vi "FPGA.vi"() -> ()   [LabVIEW 2015]
doc: "This is the primary FPGA VI for the Build Your Own Embedded System project."
uses:
  Custom Controls/Battery State.ctl
  Custom Controls/Display State.ctl
  <vilib>/Platform/TimedLoop/XDataNode/timing_clust.ctl
  <vilib>/Platform/TimedLoop/XDataNode/nitl_modes.ctl
  <vilib>/Platform/TimedLoop/XDataNode/wakeup.ctl
  <vilib>/rvi/FXPMathLib/FxpDiv/subVIs/nifxpmath_Div_SimConfig.ctl
  <vilib>/rvi/Emulation/niFpgaGetClockAttributes.vi
  <vilib>/rvi/Emulation/niFpgaSctlEmulationGetInTimedLoop.vi
  <vilib>/rvi/Emulation/niFpgaEmulationReportErrorSimple.vi
  <vilib>/EmbeddedDisplay/Hitachi HD44780/FPGA/Internal/LCD Command.vi
  <vilib>/EmbeddedDisplay/Hitachi HD44780/FPGA/Public/Command Handler (8 Bits).vi
  <vilib>/rvi/Emulation/niFpgaProcessEmulError.vi
  <vilib>/rvi/Emulation/niFpgaCriticalErrorInLSC.vi
  <vilib>/rvi/eio/common/nirviEmuTemplateMethod_errors.vi
  <vilib>/rvi/Analysis/common/codeGenErrors/XNode/niFpgaXNodeCodeGenErrorHandle.vi
  <vilib>/rvi/Analysis/utilities/niFPGA Threshold Crossing Logic.vi
  <vilib>/rvi/FXPMathLib/FxpDiv/simVIs/DllFxpDivTemp_sub.vi
  <vilib>/eio/EIONode/EIONode.xnode
  <vilib>/rvi/Analysis/measure/period/templates/niFPGA Period Edge Direction.ctl
  <vilib>/rvi/Analysis/measure/period/XNode/niFpgaAnalogPeriod.xnode
  <vilib>/Platform/TimedLoop/XDataNode/XDataNode.xnode
  <vilib>/rvi/FXPMathLib/FxpDiv/XNode/nifxpmath_Div.xnode
  <vilib>/EmbeddedDisplay/Hitachi HD44780/FPGA/HD44780 FPGA.lvlib
  <vilib>/Platform/TimedLoop/XDataNode/XDNodeRunTimeDep.lvlib
panel:
  out "FPGA Display Command":T1=enum."RPM"
  out "Battery State":T2
  in  "Max Temp":fxp<+/-,32,13>
  out "Voltage":fxp<+/-,24,5>
  out "RPM":fxp<+,32,16>
  out "Temp":fxp<+/-,32,13>
  out "Temp Warning":bool
  in  "LCD Command":T3={"device index (-1)"=-1, "operation (0)"=0}
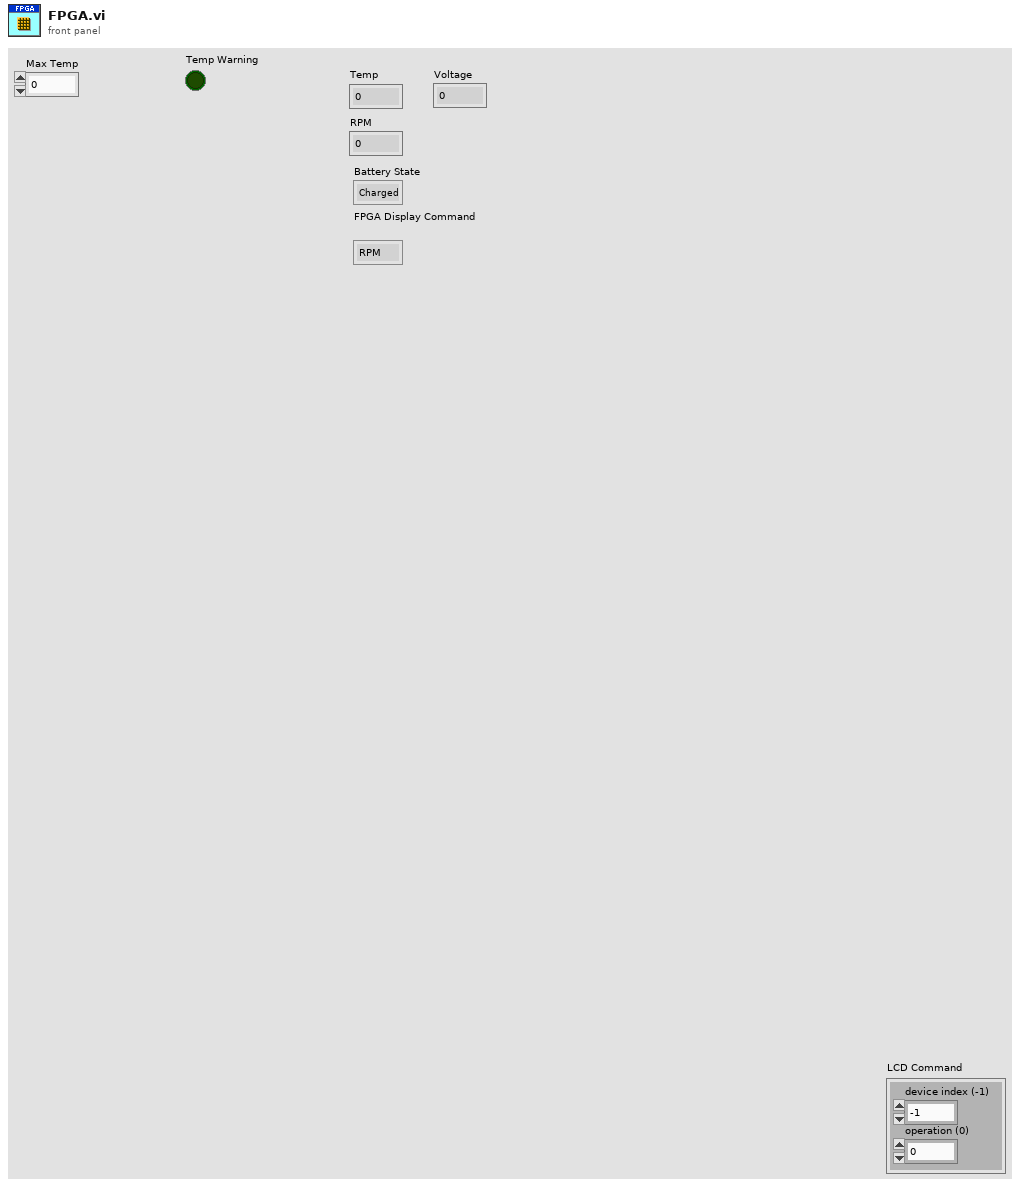
[diagram p1: front panel]
types:
  T1 = typedef "Display State.ctl" = enum16{"Battery State", "RPM", "Temp", "Voltage"}
  T2 = typedef "Battery State.ctl" = enum16{"Charged", "Running", "Low Batt"}
  T3 = cluster{"device index (-1)":i8, "operation (0)":u32}
  T4 = typedef "XDNodeRunTimeDep.lvlib/timing_clust.ctl" = cluster{"Expected End [f-1]":u64, "Actual End [f-1]":u64, "Finished Late? [f-1]":bool, "Expected End [i-1]":u64, "Actual End [i-1]":u64, "Finished Late? [i-1]":bool, "Expected Start [i]":u64, "Actual Start [i]":u64, "Expected Start [f]":u64, "Actual Start [f]":u64, "Source Name":string, "Structure Name":string, "Period":i64, "Deadline":i64, "Offset":i64, "Start":i64, "Priority":i32, "Timeout":i32, "Mode":T5, "Wakeup Reason":T6, "Error":errorcluster, "Source Type":string, "Secondary Source Type":string, "Global End Time":u64, "Global Start Time":u64, "Frame Duration":u64, "Iteration Duration":u64, "Assigned CPU":i32, "I/O Scan Engine Mode":u32}
  T5 = typedef "XDNodeRunTimeDep.lvlib/nitl_modes.ctl" = enum32{"No Change", "Process missed periods, maintain original phase", "Discard missed periods, maintain original phase", "Process missed periods, ignore original phase", "Discard missed periods, ignore original phase"}
  T6 = typedef "XDNodeRunTimeDep.lvlib/wakeup.ctl" = enum32{"Normal", "Aborted", "Asynchronous wakeup", "Timing source error", "Timed loop error", "Timeout"}
  T7 = cluster{"RS":refnum<k21>, "R/W":refnum<k21>, "E1":refnum<k21>, "E2":refnum<k21>, "DB0":refnum<k21>, "DB1":refnum<k21>, "DB2":refnum<k21>, "DB3":refnum<k21>, "DB4":refnum<k21>, "DB5":refnum<k21>, "DB6":refnum<k21>, "DB7":refnum<k21>}
  T8 = typedef "HD44780 Common.lvlib/lcd command cluster.ctl" = cluster{"device index (-1)":i8, "operation (0)":u32}
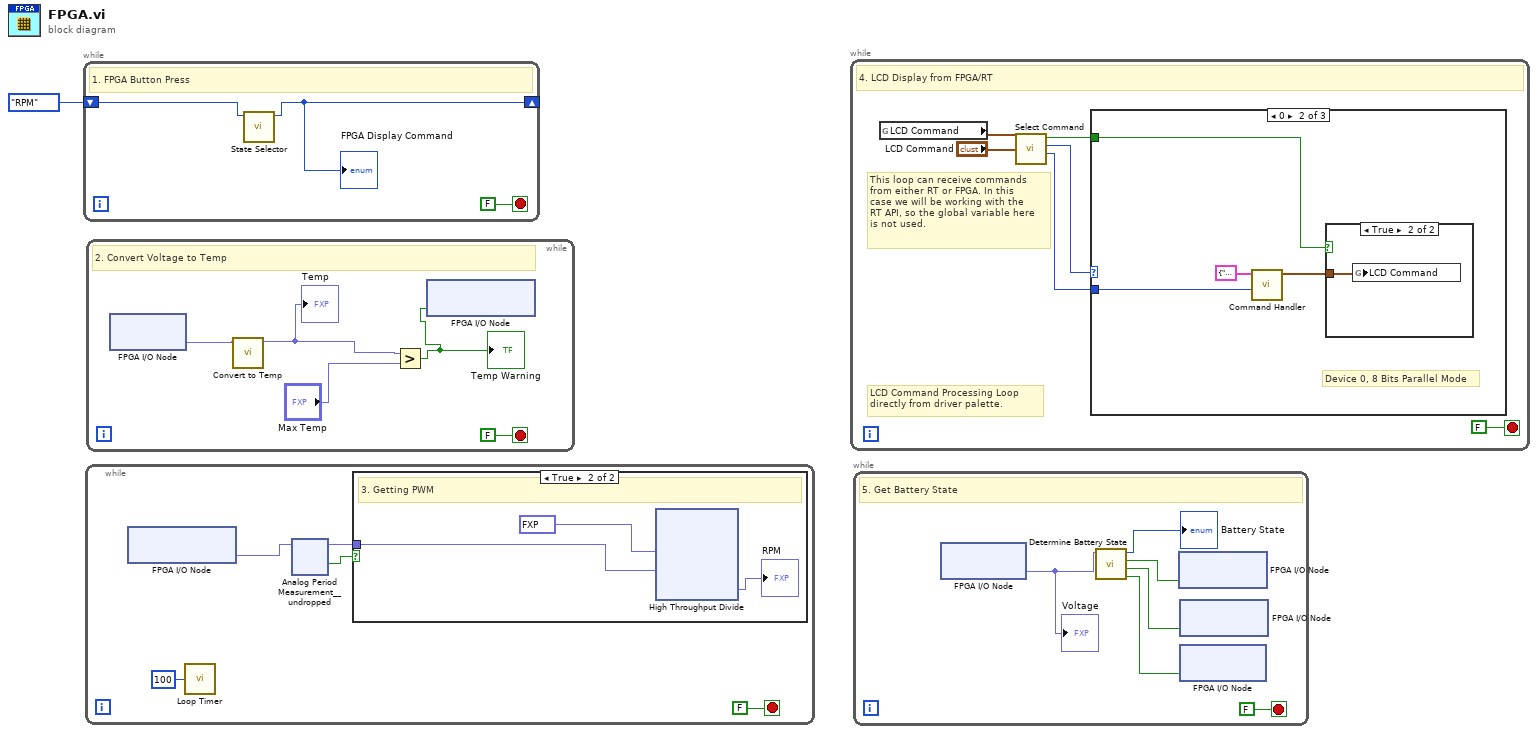
[diagram p0: block diagram]
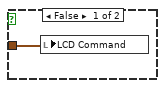
[diagram p4: hidden frame]
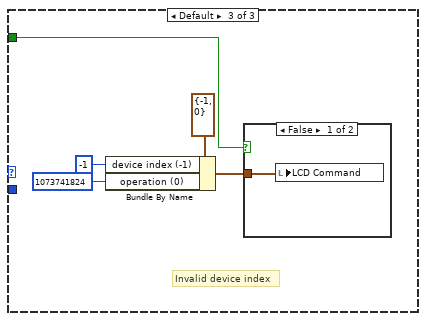
[diagram p5: hidden frame]
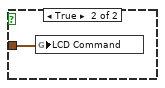
[diagram p6: hidden frame]
diagram:
  n1 = while {
    shift-right: [w2] -> _
    shift-left: Display_State."RPM" ("Enum") -> [w3]
    stop <- FALSE stop-if-true
    # "1. FPGA Button Press"
    n2 = call "State Selector.vi"("Display State In"=w3) -> ("Display State Out"=w2:T1)  [unwired: 9 in, 1 out]
    "FPGA Display Command" <- w2
  }
  n3 = while {
    stop <- FALSE stop-if-true
    n4 = xnode "FPGA I/O Node"() -> ("EnginePWM"=w7:fxp<+/-,24,5>)  [unwired: 1 in, 1 out]
    n5 = call "Loop Timer"("Count(uSec)"=u32 100 ("Count(Ticks)")) -> ()  [unwired: 1 out]
    n6 = xnode "Analog Period Measurement__undropped"("input data"=w7) -> ("period (samples)"=w5:fxp<+,32,16>, "output valid"=w6:bool)  [unwired: 4 in, 2 out]
    n7 = case shown="True" w6 {
      tunnel: w5 -> [_ w11]
      frame False {
      }
      frame True {
        # "3. Getting PWM"
        n8 = xnode "High Throughput Divide"("x"=fxp<+,32,32> 10000.0, "y"=w11) -> ("x/y"=→"RPM":fxp<+,32,16>)
      }
    }
  }
  n9 = while {
    stop <- FALSE stop-if-true
    # "2. Convert Voltage to Temp"
    n10 = xnode "FPGA I/O Node"() -> ("Temp"=w160:fxp<+/-,24,5>)  [unwired: 1 in, 1 out]
    n11 = call "Convert to Temp.vi"("Voltage"=w160) -> ("deg C"=w157:fxp<+/-,32,13>)  [unwired: 10 in]
    "Temp" <- w157
    n12 = Greater?(x=w157, y="Max Temp") -> (0:w159:bool)
    "Temp Warning" <- w159
    n13 = xnode "FPGA I/O Node"("LEDWarning"=w159) -> ()  [unwired: 1 in, 1 out]
  }
  n14 = while {
    stop <- FALSE stop-if-true
    # "4. LCD Display from FPGA/RT"
    # "This loop can receive commands\nfrom either RT or FPGA. In this\ncase we will be working with the \nRT API, so the global variable here\nis not used."
    # "LCD Command Processing Loop\ndirectly from driver palette."
    n15 = global read "LCD Command.vi" "LCD Command"() -> (w162:T8)
    n16 = call <vilib>:"Select Command.vi"("Host LCD Command"="LCD Command", "FPGA LCD Command"=w162) -> ("operation"=w164:u32, "device index"=w165:i8, "FPGA? True : False"=w163:bool)  [unwired: 7 in]
    n17 = case shown="0" w165 {
      tunnel: w164 -> [_ w171 _]
      tunnel: w163 -> [_ w170 w178]
      frame -1 {
        # "IDLE State"
      }
      frame 0 {
        # "Device 0, 8 Bits Parallel Mode"
        n18 = call-poly <vilib>:"Command Handler.vi"("operation"=w171, "device connection map in"=T7 {"RS"="DIO19", "R/W"="DIO18", "E1"="DIO17", "E2"="DIO17", "DB0"="DIO20", "DB1"="DIO21", "DB2"="DIO22", "DB3"="DIO23", "DB4"="DIO24", "DB5"="DIO25", "DB6"="DIO26", "DB7"="DIO27"}) -> ("result"=w169:T8)  [unwired: 9 in]
        n19 = case shown="True" w170 {
          tunnel: w169 -> [w172 w173]
          frame False {
            n20 = local write "LCD Command"(w172) -> ()
          }
          frame True {
            n21 = global write "LCD Command.vi" "LCD Command"(w173) -> ()
          }
        }
      }
      frame Default {
        # "Invalid device index"
        n22 = Bundle By Name(cluster=T3 {"device index (-1)"=-1, "operation (0)"=0} ("LCD Command"), "device index (-1)"=i8 -1 ("LCD_device index (-1)"), "operation (0)"=u32 1073741824 ("LCD_operation (0)")) -> (w174:T3)
        n23 = case shown="False" w178 {
          tunnel: w174 -> [w179 w180]
          frame False {
            n24 = local write "LCD Command"(w179) -> ()
          }
          frame True {
            n25 = global write "LCD Command.vi" "LCD Command"(w180) -> ()
          }
        }
      }
    }
  }
  n26 = while {
    stop <- FALSE stop-if-true
    # "5. Get Battery State"
    n27 = xnode "FPGA I/O Node"() -> ("BattVolt"=w181:fxp<+/-,24,5>)  [unwired: 1 in, 1 out]
    "Voltage" <- w181
    n28 = call "Determine Battery State.vi"("Voltage"=w181) -> ("Low Battery"=w182:bool, "Running"=w183:bool, "Fully Charged"=w184:bool, "Battery State"=→"Battery State":T2)  [unwired: 7 in]
    n29 = xnode "FPGA I/O Node"("Charged"=w184) -> ()  [unwired: 1 in, 1 out]
    n30 = xnode "FPGA I/O Node"("Running"=w183) -> ()  [unwired: 1 in, 1 out]
    n31 = xnode "FPGA I/O Node"("LowBatt"=w182) -> ()  [unwired: 1 in, 1 out]
  }
